vi "Set Parameters GUI.vi"(8 "error in (no error)":errorcluster, 11 "Lakeshore 325 in":refnum<class "Lakeshore 325.lvclass">) -> (0 "error out":errorcluster, 3 "Lakeshore 325 out":refnum<class "Lakeshore 325.lvclass">)   [LabVIEW 2022 SP3, in "Lakeshore 325.lvclass"]
uses:
  Lakeshore 325.lvclass
  Lakeshore 325.lvclass/Lakeshore 325.ctl
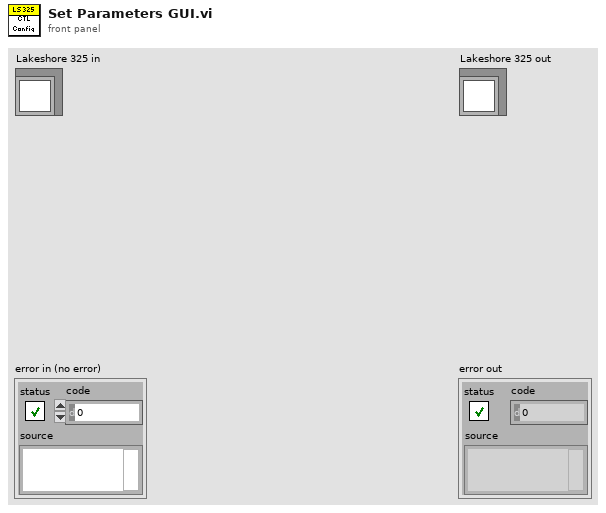
[diagram p1: front panel]
types:
  T1 = typedef "Temp Control.lvclass/Temp Control Parameters.ctl" = cluster{"Mode":u16, "Setpoint":dbl, "Manual Power (%)":dbl, "Control Parameters":cluster{"P":dbl, "I":dbl, "D":u16}, "Heater Range":u16, "Default Range":u16}
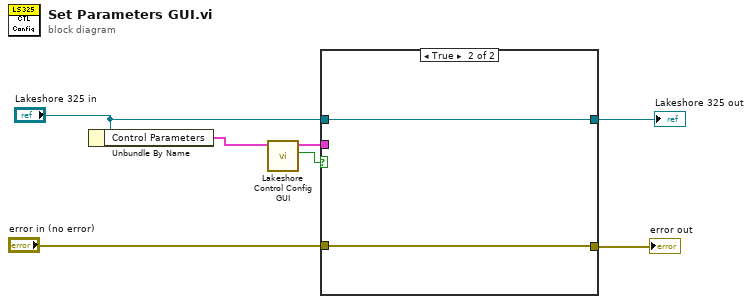
[diagram p0: block diagram]
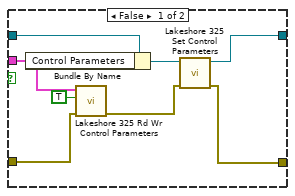
[diagram p2: hidden frame]
diagram:
  n1 = Unbundle By Name("Lakeshore 325 in") -> ("Control Parameters"=w7:T1)
  n2 = call "Lakeshore Control Config GUI.vi"("Control Parameters"=w7) -> ("cancelled"=w6:bool, "Temp Control Parms out"=w3:T1)  [unwired: 9 in]
  n3 = case shown="True" w6 {
    tunnel: [w11 w17] -> w5
    tunnel: "Lakeshore 325 in" -> [w15 w17]
    tunnel: w3 -> [w14 _]
    tunnel: "error in (no error)" -> [w9 w16]
    tunnel: [w8 w16] -> w1
    frame False {
      n4 = Bundle By Name(cluster=w15, "Control Parameters"=w14) -> (w12:refnum<class "Lakeshore 325.lvclass">)
      n5 = call "Lakeshore 325 Rd Wr Control Parameters.vi"("error in (no error)"=w9, "Write? (F:Read)"=TRUE, "Control Parameters"=w14) -> ("error out"=w10:errorcluster)  [unwired: 7 in, 1 out]
      n6 = call "Lakeshore 325 Set Control Parameters.vi"("error in (no error)"=w10, "Lakeshore 325 in"=w12) -> ("error out"=w8:errorcluster, "Lakeshore 325 out"=w11:refnum<class "Lakeshore 325.lvclass">)  [unwired: 8 in]
    }
    frame True {
    }
  }
  "error out" <- w1
  "Lakeshore 325 out" <- w5
